vi "AutoSetPreSetPos.vi"(8 "error in (no error)":errorcluster, 10 "Game Piece":T1, 11 "Position":T2=enum."Middle") -> (0 "error out":errorcluster)   [LabVIEW 2023]
uses:
  Arm/ArmPositionPreset.ctl
  Arm/ArmGamePiecePreset.ctl
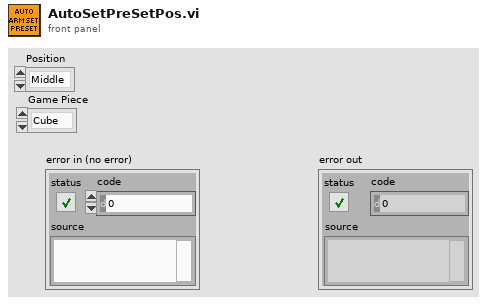
[diagram p1: front panel]
types:
  T1 = typedef "ArmGamePiecePreset.ctl" = enum16{"Cube", "Cone"}
  T2 = typedef "ArmPositionPreset.ctl" = enum16{"Upper", "Lower", "Middle", "Home", "Shelf", "Floor", "HalfFloor", "HalfHome"}
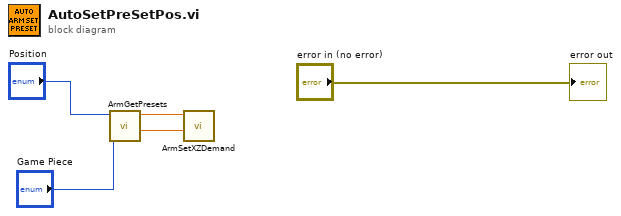
[diagram p0: block diagram]
diagram:
  n1 = call "ArmGetPresets.vi"("Game Piece"="Game Piece", "Position"="Position") -> ("z"=w3:dbl, "x"=w4:dbl)  [unwired: 8 in]
  n2 = call "ArmSetXZDemand.vi"("SetZ"=w3, "SetX"=w4) -> ()  [unwired: 10 in]
  "error out" <- "error in (no error)"
